vi "getState.vi"(8 "error in (no error)":errorcluster, 11 "SettingUpState in":refnum<class "SettingUpState.lvclass">) -> (0 "error out":errorcluster, 2 "DeviceStatus":T1, 3 "SettingUpState out":refnum<class "SettingUpState.lvclass">)   [LabVIEW 2016, in "SettingUpState.lvclass"]
uses:
  SettingUpState.lvclass
  Typedefs/DeviceStatus.ctl
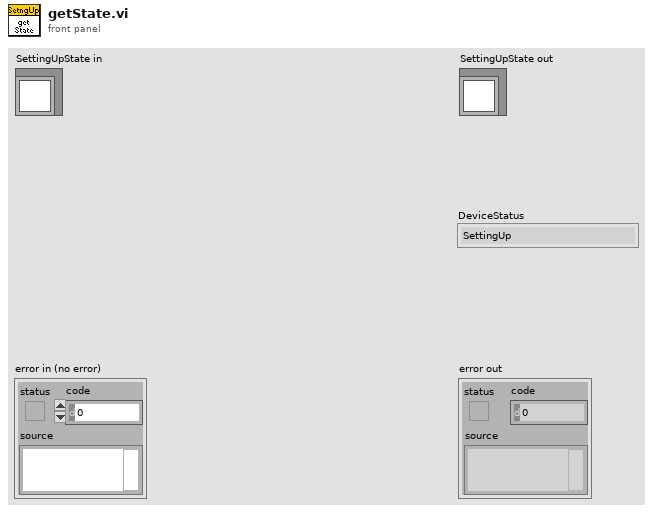
[diagram p1: front panel]
types:
  T1 = typedef "DeviceStatus.ctl" = enum16{"SettingUp", "Ready", "Offline", "Fault"}
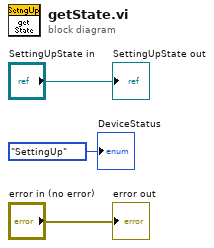
[diagram p0: block diagram]
diagram:
  "error out" <- "error in (no error)"
  "SettingUpState out" <- "SettingUpState in"
  "DeviceStatus" <- DeviceStatus."SettingUp" ("DeviceStatus")
